vi "sort.volumes.vi"(11 "volumes":T1[](array[typedef])) -> (1 "end date":timestamp, 2 "start date":timestamp, 3 "volumes by row":cluster{"Array":T1[]}[](array[cluster]))   [LabVIEW 2024]
uses:
  volume.object--cluster.ctl
  definitions/volume.type--enum.ctl
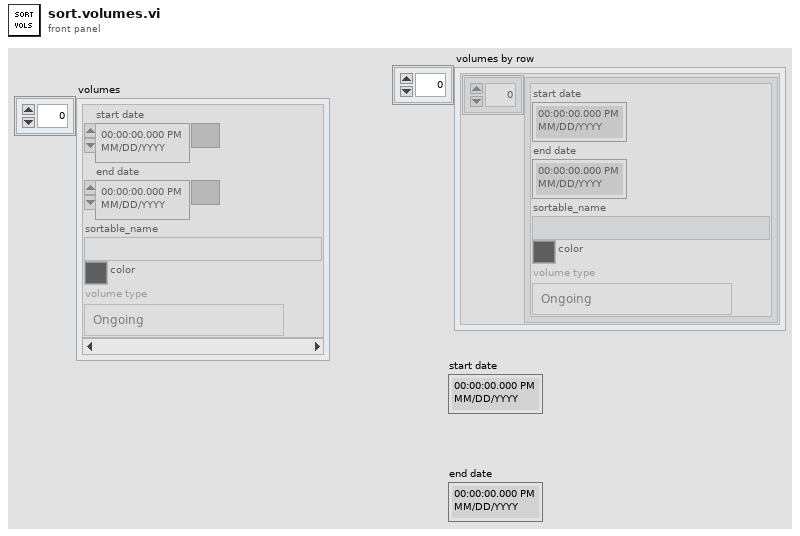
[diagram p1: front panel]
types:
  T1 = typedef "volume.object--cluster.ctl" = cluster{"start date":timestamp, "end date":timestamp, "sortable_name":string, "color":u32, "volume type":T2}
  T2 = typedef "volume.type--enum.ctl" = enum16{"Ongoing", "Limited Series", "Annual", "One Shot", "Reprint/Document"}
  T3 = cluster{"open start":timestamp, "open end":timestamp}
  T4 = cluster{"open start":timestamp, "open end":timestamp}[]
  T5 = cluster{T1[], cluster{"open start":timestamp, "open end":timestamp}[]}
  T6 = cluster{T1[], cluster{"open start":timestamp, "open end":timestamp}[]}[]
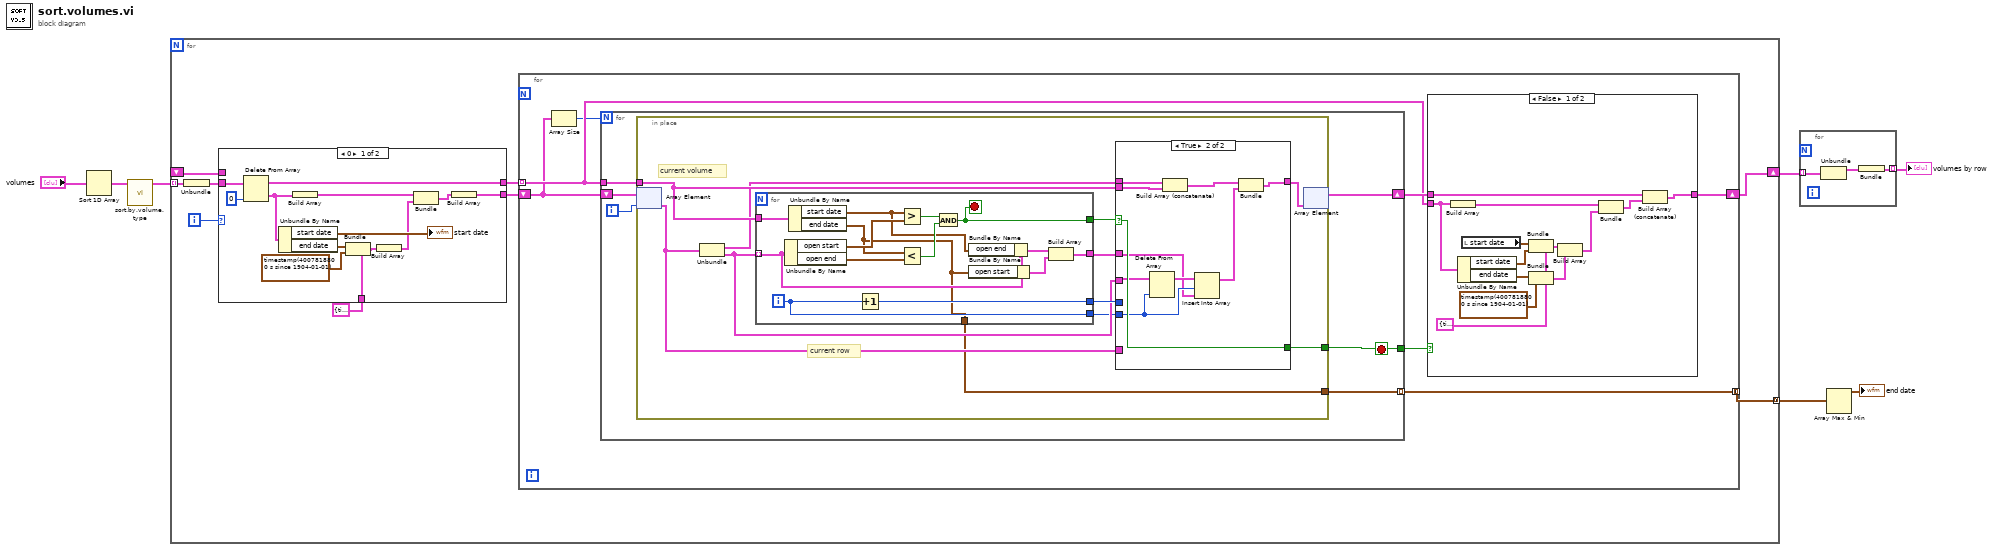
[diagram p0: block diagram]
diagram:
  n1 = Sort 1D Array(array="volumes") -> (sorted array=w4:T1[])
  n2 = call "sort.by.volume.type.vi"("Array in"=w4) -> ("Array"=w3:cluster{T1[]}[])  [unwired: 10 in]
  n3 = for {
    tunnel: [w14] -> w6 mode=concatenating
    tunnel: w3 -> [w13] mode=indexing
    shift-right: [w11] -> w2
    shift-left: _ -> [w9]
    i -> [w10]
    n4 = Unbundle(w13) -> (w12:T1[])
    n5 = case shown="0" w10 {
      tunnel: [w28 w30] -> w16
      tunnel: [w25 w31] -> w15
      tunnel: w12 -> [w24 w30]
      tunnel: w9 -> [_ w31]
      tunnel: T3 {"open start"=timestamp(0 s since 1904-01-01), "open end"=timestamp(0 s since 1904-01-01)} -> [w18 _]
      frame 0 {
        n6 = Delete From Array(array=w24, index=0) -> (deleted portion=w23:T1, array with subset deleted=w28:T1[])  [unwired: 1 in]
        n7 = Unbundle By Name(w23) -> ("start date"=→"start date":timestamp, "end date"=w21:timestamp)
        n8 = Build Array(w23) -> (w27:T1[])
        n9 = Bundle(cluster=w18, "open start"=w21, "open end"=timestamp(4007818800 s since 1904-01-01) ("current time")) -> (w19:T3)
        n10 = Build Array(w19) -> (w20:T4)
        n11 = Bundle(w27, w20) -> (w26:T5)  [unwired: 1 in]
        n12 = Build Array(w26) -> (w25:T6)
      }
      frame Default {
      }
    }
    n13 = for {
      tunnel: w16 -> [w35] mode=indexing
      shift-right: [w36] -> w11
      shift-left: w15 -> [w34]
      tunnel: [w32] -> w14 mode=concatenating
      n14 = Array Size(array=w34) -> (size(s)=w33:i32)
      n15 = for {
        N: w33 -> [_]
        tunnel: w35 -> [w58]
        shift-right: [w56] -> w37
        shift-left: w34 -> [w57]
        tunnel: [w55] -> w38
        tunnel: [w54] -> w32 mode=indexing
        i -> [w53]
        stop <- w55 stop-if-true
        n16 = in-place {
          in-place-border: [w69] -> w55
          in-place-border: w58 -> [w66]
          in-place-border: [w59] -> w54
          # "current row"
          # "current volume"
          n17 = in-place-array #1(w57, w53) -> (w67:T5)
          n18 = Unbundle(w67) -> (w64:T1[], w62:T4)
          n19 = for {
            tunnel: w66 -> [w83]
            tunnel: [w79] -> w65
            tunnel: [w72] -> w63
            tunnel: w62 -> [w77] mode=indexing
            tunnel: [w76] -> w60
            tunnel: [w75] -> w61
            tunnel: [w70] -> w59
            i -> [w75]
            stop <- w79 stop-if-true
            n20 = Unbundle By Name(w77) -> ("open start"=w78:timestamp, "open end"=w82:timestamp)
            n21 = Unbundle By Name(w83) -> ("start date"=w71:timestamp, "end date"=w70:timestamp)
            n22 = Increment(x=w75) -> (x+1=w72:i32)
            n23 = Greater?(x=w71, y=w78) -> (0:w81:bool)
            n24 = Less?(x=w70, y=w82) -> (x < y?=w80:bool)
            n25 = And(x=w81, y=w80) -> (x .and. y?=w79:bool)
            n26 = Bundle By Name(cluster=w77, "open end"=w71) -> (w74:T3)
            n27 = Bundle By Name(cluster=w77, "open start"=w70) -> (w73:T3)
            n28 = Build Array(w74, w73) -> (w76:T4)
          }
          n29 = case shown="True" w65 {
            selector: w65 -> [w84 w95]
            tunnel: [w84 w95] -> w69
            tunnel: w64 -> [_ w93]
            tunnel: w66 -> [_ w92]
            tunnel: [w85 w94] -> w68
            tunnel: w67 -> [w85 _]
            tunnel: w63 -> [_ _]
            tunnel: w62 -> [_ w90]
            tunnel: w61 -> [_ w88]
            tunnel: w60 -> [_ w87]
            frame False {
            }
            frame True {
              n30 = Delete From Array(array=w90, index=w88) -> (array with subset deleted=w89:T4)  [unwired: 1 in, 1 out]
              n31 = Build Array (concatenate)(w93, w92) -> (w91:T1[])
              n32 = Insert Into Array(array=w89, index=w88, new element=w87) -> (w86:T4)
              n33 = Bundle(w91, w86) -> (w94:T5)  [unwired: 1 in]
            }
          }
          n34 = in-place-array #1(w68) -> (w56:T6)  [unwired: 1 out]
        }
      }
      n35 = case shown="False" w38 {
        tunnel: [w50 w52] -> w36
        tunnel: w37 -> [w51 w52]
        tunnel: w35 -> [w45 _]
        frame False {
          w42 = T3 {"open start"=timestamp(0 s since 1904-01-01), "open end"=timestamp(0 s since 1904-01-01)}
          n36 = Build Array(w45) -> (w49:T1[])
          n37 = Unbundle By Name(w45) -> ("start date"=w44:timestamp, "end date"=w41:timestamp)
          n38 = local read "start date"() -> (w46:timestamp)
          n39 = Bundle(cluster=w42, "open start"=w46, "open end"=w44) -> (w43:T3)
          n40 = Bundle(cluster=w42, "open start"=w41, "open end"=timestamp(4007818800 s since 1904-01-01) ("current time")) -> (w39:T3)
          n41 = Build Array(w43, w39) -> (w48:T4)
          n42 = Bundle(w49, w48) -> (w47:T5)  [unwired: 1 in]
          n43 = Build Array (concatenate)(w51, w47) -> (w50:T6)
        }
        frame True {
        }
      }
    }
  }
  n44 = for {
    tunnel: w2 -> [w98] mode=indexing
    tunnel: [w96] -> w1 mode=indexing
    n45 = Unbundle(w98) -> (w97:T1[])  [unwired: 1 out]
    n46 = Bundle(w97) -> (w96:cluster{T1[]})  [unwired: 1 in]
  }
  "volumes by row" <- w1
  n47 = Array Max & Min(array=w6) -> (max value=→"end date":timestamp)  [unwired: 3 out]
